vi "testParseTopicString.vi"(8 "error in (no error)":errorcluster) -> (0 "error out":errorcluster)   [LabVIEW 2018]
uses:
  SALTypeGenerator/Topic/Topic.lvclass
  SALTypeGenerator/ElementFactory/ElementFactory/ElementFactory.lvclass
  home/teweitsai/Documents/github/ts_SALLabVIEW/SALTypeGenerator/ElementFactory/IElementFactory/IElementFactory.lvclass
  SALTypeGenerator/Elements/Array/Array.lvclass
  SALTypeGenerator/Topic/Topic.lvclass/Topic.ctl
  SALTypeGenerator/Elements/Array/Array.lvclass/Array.ctl
  <vilib>/addons/_JKI Toolkits/Caraya/classes/Assert/Assert Equal Value_Variant.vi
  SALTypeGenerator/Element/Element.lvclass
  <vilib>/addons/_JKI Toolkits/Caraya/classes/Test/Test.lvclass
  <vilib>/addons/_JKI Toolkits/Caraya/classes/Assert/Assert.lvclass
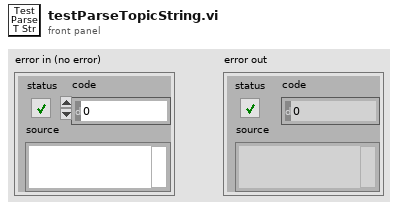
[diagram p1: front panel]
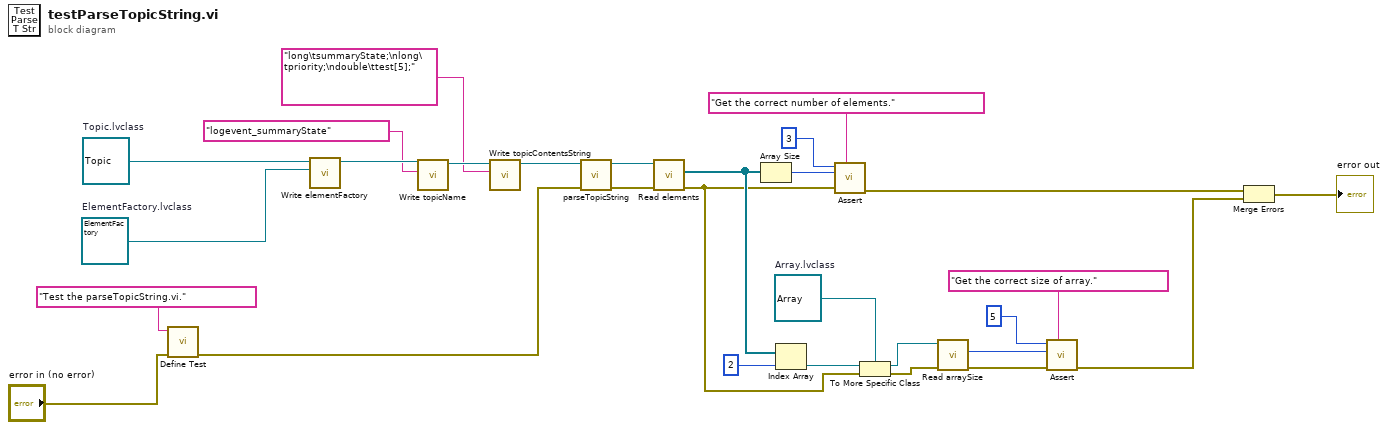
[diagram p0: block diagram]
diagram:
  w11 = refnum<class "Array.lvclass"> refnum  # Array.lvclass
  w28 = refnum<class "ElementFactory.lvclass"> refnum  # ElementFactory.lvclass
  w29 = refnum<class "Topic.lvclass"> refnum  # Topic.lvclass
  n1 = call <vilib>:"Define Test.vi"("error in (no error)"="error in (no error)", "Label (VI Title)"="Test the parseTopicString.vi.") -> ("error out"=w18:errorcluster)  [unwired: 9 in]
  n2 = call "Write elementFactory.vi"("IElementFactory.lvclass"=w28, "Topic in"=w29) -> ("Topic out"=w27:refnum<class "Topic.lvclass">)  [unwired: 9 in]
  n3 = call "Write topicName.vi"("topicName"="logevent_summaryState", "Topic in"=w27) -> ("Topic out"=w26:refnum<class "Topic.lvclass">)  [unwired: 9 in]
  n4 = call "Write topicContentsString.vi"("topicContentsString"="long\tsummaryState;\nlong\tpriority;\ndouble\ttest[5];", "Topic in"=w26) -> ("Topic out"=w25:refnum<class "Topic.lvclass">)  [unwired: 9 in]
  n5 = call "parseTopicString.vi"("error in (no error)"=w18, "Topic in"=w25) -> ("error out"=w21:errorcluster, "Topic out"=w22:refnum<class "Topic.lvclass">)  [unwired: 8 in]
  n6 = call "Read elements.vi"("error in (no error)"=w21, "Topic in"=w22) -> ("error out"=w9:errorcluster, "elements"=w14:refnum<class "Element.lvclass">[])  [unwired: 7 in, 1 out]
  n7 = Array Size(array=w14) -> (size(s)=w17:i32)
  n8 = Index Array(array=w14, index=2) -> (element=w12:refnum<class "Element.lvclass">)
  n9 = call-poly <vilib>:"Assert.vi"("Label"="Get the correct number of elements.", "error in (no error)"=w9, "Y"=w17, "X"=3) -> ("error out"=w3:errorcluster)  [unwired: 7 in]
  n10 = To More Specific Class(target class=w11, reference=w12, error in=w9) -> (specific class reference=w10:refnum<class "Array.lvclass">, error out=w8:errorcluster)
  n11 = call "Read arraySize.vi"("error in (no error)"=w8, "Array in"=w10) -> ("error out"=w7:errorcluster, "arraySize"=w6:u16)  [unwired: 7 in, 1 out]
  n12 = call-poly <vilib>:"Assert.vi"("Label"="Get the correct size of array.", "error in (no error)"=w7, "Y"=w6, "X"=5) -> ("error out"=w2:errorcluster)  [unwired: 7 in]
  n13 = Merge Errors(w3, w2) -> (→"error out":errorcluster)
